vi "XCAN_PDO_Enable_&_Disable.vi"() -> ()   [LabVIEW 2016]
uses:
  <vilib>/Stratom, Inc/X-Modules for myRIO/Type Defs/MXPChannel.ctl
  <vilib>/Stratom, Inc/X-CAN for myRIO (API)/X-CAN Class/Type Definitions/CAN_Speed.ctl
  <vilib>/Stratom, Inc/X-CAN for myRIO (API)/X-CAN Class/Type Definitions/CANFrame.ctl
  <vilib>/myRIO/Common/Instrument Driver Framework/myRIO v1.0/UART/vis/myRIO v1.0 Close UART.vi
  <vilib>/myRIO/Common/Instrument Driver Framework/Utilities/vis/FPGA Ref Manager.vi
  <vilib>/myRIO/Common/Instrument Driver Framework/myRIO v1.0/myRIO v1.0 Reset FPGA.vi
  <vilib>/myRIO/Common/Instrument Driver Framework/myRIO v1.0/IRQ/vis/myRIO v1.0 IRQ Info FGV.vi
  <vilib>/myRIO/Common/Instrument Driver Framework/myRIO v1.0/IRQ/vis/myRIO v1.0 Timer IRQ Info FGV.vi
  <vilib>/myRIO/Common/Instrument Driver Framework/myRIO v1.0/IRQ/vis/myRIO v1.0 ISR Agent.vi
  <vilib>/Stratom, Inc/X-CAN for myRIO (API)/X-CAN Class/X-CAN.lvclass
  <vilib>/myRIO/Instrument Drivers/Utilities/Utilities.lvlib
panel:
  in  "Enable / Disable PDO":bool
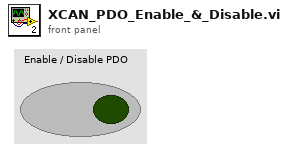
[diagram p1: front panel]
types:
  T1 = typedef "X-CAN.lvclass/CAN_Speed.ctl" = u8
  T2 = typedef "MXPChannel.ctl" = enum16{"A/MXP", "B/MXP"}
  T3 = typedef "X-CAN.lvclass/CANFrame.ctl" = cluster{"identifier":u32, "extended?":bool, "echo?":bool, "payload":u8[], "timestamp":timestamp}
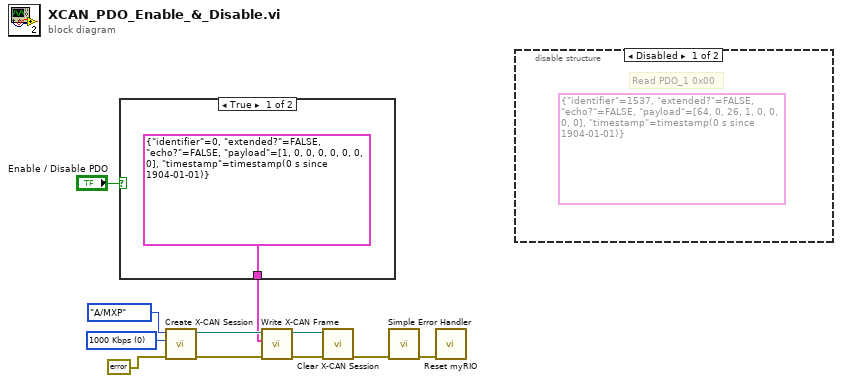
[diagram p0: block diagram]
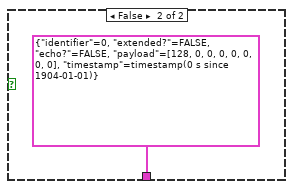
[diagram p3: hidden frame]
diagram:
  w8 = T1 0 items=["125 Kbps"=7, "250 Kbps"=3, "500 Kbps"=1, "1000 Kbps"=0, "95.238 Kbps"=6] ("CAN Speed [Kbps]")
  n1 = case shown="True" "Enable / Disable PDO" {
    tunnel: [T3 {"identifier"=0, "extended?"=FALSE, "echo?"=FALSE, "payload"=[1, 0, 0, 0, 0, 0, 0, 0], "timestamp"=timestamp(0 s since 1904-01-01)} ("CAN Frame") T3 {"identifier"=0, "extended?"=FALSE, "echo?"=FALSE, "payload"=[128, 0, 0, 0, 0, 0, 0, 0], "timestamp"=timestamp(0 s since 1904-01-01)} ("CAN Frame")] -> w6
    frame True {
    }
    frame False {
    }
  }
  n2 = call <vilib>:"Create X-CAN Session.vi"("error in (no error)"=errorcluster {"status"=FALSE, "code"=0, "source"=""}, "CAN Speed [Kbps]"=w8, "MXP Channel"=MXPChannel."A/MXP") -> ("error out"=w11:errorcluster, "X-CAN Session out"=w10:refnum<class "X-CAN.lvclass">)  [unwired: 7 in]
  n3 = call <vilib>:"Write X-CAN Frame.vi"("error in"=w11, "CAN Frame"=w6, "X-CAN Session in"=w10) -> ("error out"=w2:errorcluster, "X-CAN Session out"=w3:refnum<class "X-CAN.lvclass">)  [unwired: 7 in]
  n4 = call <vilib>:"Clear X-CAN Session.vi"("error in (no error)"=w2, "X-CAN Session in"=w3) -> ("error out"=w5:errorcluster)  [unwired: 9 in]
  n5 = call <vilib>:"Simple Error Handler.vi"("error in (no error)"=w5) -> ("error out"=w4:errorcluster)  [unwired: 4 in, 4 out]
  n6 = call <vilib>:"Reset myRIO.vi"("error in (no error)"=w4) -> ()  [unwired: 10 in, 1 out]
  n7 = disable-structure shown="Disabled" {
    frame Disabled {
      (unwired) T3 {"identifier"=1537, "extended?"=FALSE, "echo?"=FALSE, "payload"=[64, 0, 26, 1, 0, 0, 0, 0], "timestamp"=timestamp(0 s since 1904-01-01)} ("CAN Frame")
      # "Read PDO_1 0x00"
    }
    frame Enabled {
    }
  }
